vi "sub_simluation_q.vi"(7 "cmd":enum16{"create", "write", "read", "close"}(ring), 8 "error in":errorcluster, 11 "data":enum16{"run", "stop"}(ring)) -> (0 "error out":errorcluster, 3 "queue out":refnum<queue>)   [LabVIEW 2016]
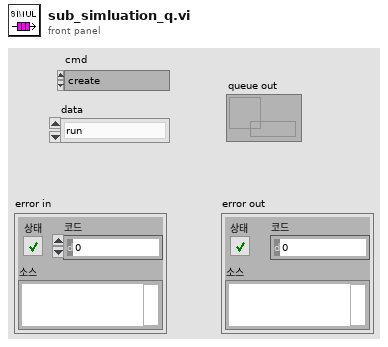
[diagram p1: front panel]
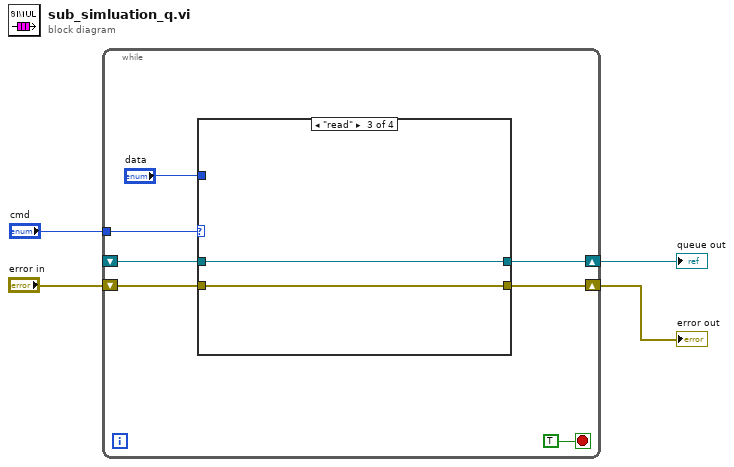
[diagram p0: block diagram]
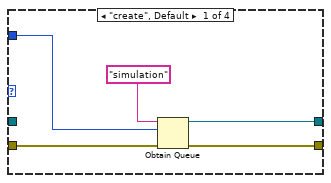
[diagram p2: hidden frame]
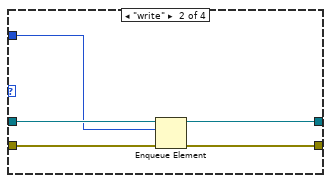
[diagram p3: hidden frame]
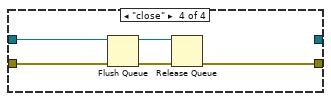
[diagram p4: hidden frame]
diagram:
  n1 = while {
    tunnel: "cmd" -> [w10]
    shift-right: [w8] -> w3
    shift-left: "error in" -> [w9]
    shift-right: [w7] -> w2
    shift-left: _ -> [w6]
    stop <- TRUE stop-if-true
    n2 = case shown="\"read\"" w10 {
      tunnel: w9 -> [w16 w21 w23 w24]
      tunnel: [w15 w20 w23 w27] -> w8
      tunnel: "data" -> [w13 w17 _ _]
      tunnel: [w12 w18 w22 _] -> w7
      tunnel: w6 -> [_ w19 w22 w25]
      frame "create", Default {
        n3 = Obtain Queue(name (unnamed)="simulation" ("이름(이름없음)"), element data type=w13, error in (no error)=w16) -> (queue out=w12:refnum<queue>, error out=w15:errorcluster)  [unwired: 2 in, 1 out]
      }
      frame "write" {
        n4 = Enqueue Element(queue=w19, element=w17, error in (no error)=w21) -> (queue out=w18:refnum<queue>, error out=w20:errorcluster)  [unwired: 1 in, 1 out]
      }
      frame "read" {
      }
      frame "close" {
        n5 = Flush Queue(queue=w25, error in (no error)=w24) -> (queue out=w26:refnum<queue>, error out=w28:errorcluster)  [unwired: 1 out]
        n6 = Release Queue(queue=w26, error in (no error)=w28) -> (error out=w27:errorcluster)  [unwired: 1 in, 2 out]
      }
    }
  }
  "error out" <- w3
  "queue out" <- w2
